vi "HMI Startup.vi"() -> ()   [LabVIEW 2019]
uses:
  <vilib>/Utility/sysdir.llb/System Directory Type.ctl
  <vilib>/NI/Current Value Table/Type Defs/Data Types.ctl
  <vilib>/NI/Current Value Table/Type Defs/Single Tag.ctl
  <vilib>/NI/STM/TCP/Read Meta Data (TCP Ref).vi
  <vilib>/NI/Current Value Table/DataTypes/Boolean_Write.vi
  <vilib>/NI/STM/TCP/Get Connection Reference (TCP).vi
  <vilib>/NI/Current Value Table/Type to Enum.vi
  <vilib>/NI/Current Value Table/DataTypes/Boolean_Type To Enum.vi
  <vilib>/NI/STM/TCP/Read Meta Data (TCP Clst).vi
  <vilib>/NI/STM/TCP/Write Message (TCP).vi
  <vilib>/NI/Current Value Table/FGVs/CVT Globals.vi
  <vilib>/NI/Current Value Table/FGVs/Tag Memory.vi
  <vilib>/NI/Current Value Table/Memory Block.vi
  <vilib>/NI/Current Value Table/DataTypes/Boolean_Memory Block.vi
  <vilib>/NI/Current Value Table/Current Value Table.lvlib
  <vilib>/NI/STM/NI STM.lvlib
panel:
  in  "Listbox":i32(listbox)=-1
  out "Sweep Time":dbl(graph)
  out "PLC Sweep Time":dbl
  out "Stop":bool
  out "PLC Firmware":string
  out "PLC Model":string
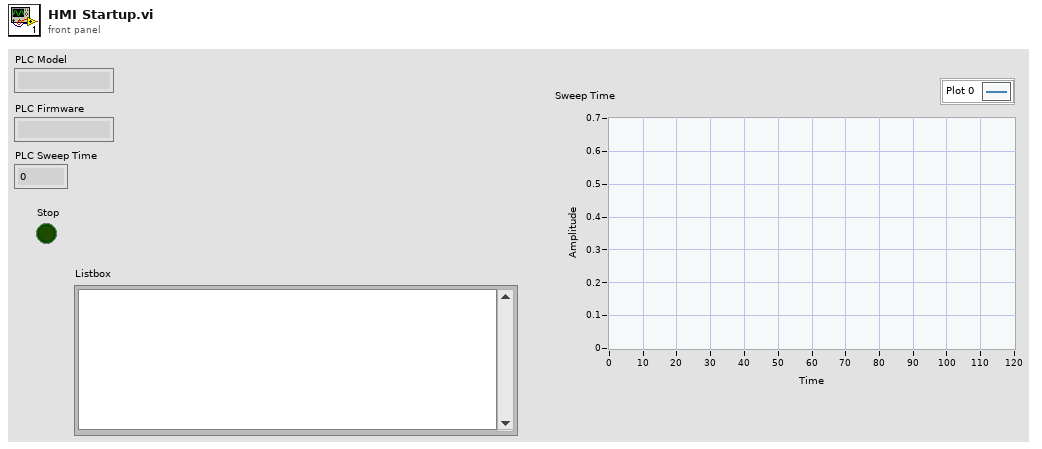
[diagram p1: front panel]
types:
  T1 = typedef "Current Value Table.lvlib/Single Tag.ctl" = cluster{"Data Type":T2, "Name":string, "Value":string, "Description":string}
  T2 = typedef "Current Value Table.lvlib/Data Types.ctl" = enum16{"Double", "Single", "I64", "I32", "I16", "I8", "U64", "U32", "U16", "U8", "String", "Boolean", "Array of U8", "Array of U16", "Array of U32", "Array of U64", "Array of I64", "Array of I32", "Array of I16", "Array of I8", "Array of Double", "Array of Single", "Array of Boolean", "Array of String"}
  T3 = typedef "System Directory Type.ctl" = i32
  T4 = typedef "tae_AlarmTagConfiguration.ctl" = cluster{"Name":string, "DataType":T5, "Alarm Configuration":T6}
  T5 = typedef "cvt_Data Types.ctl" = enum16{"Bool", "U8", "I32", "Double", "String", "Enum"}
  T6 = typedef "tae_AlarmConfiguration.ctl" = cluster{"Type":T7, "High Level":dbl, "Low Level":dbl, "Hysterisis":dbl, "Deadband":dbl}
  T7 = typedef "tae_AlarmType.ctl" = enum32{"Bool True", "Bool False", "Over Limit", "Under Limit", "Out-of-Range", "Enum Equal", "Enum Not Equal"}
  T8 = typedef "Current Value Table.lvlib/File Format.ctl" = cluster{"Tags":T1[], "Group Listings":T9[]}
  T9 = typedef "Current Value Table.lvlib/Tag Grouping set.ctl" = cluster{"Group":string, "Tag Names":string[]}
  T10 = typedef "NI STM.lvlib/TCP Connection Info.ctl" = cluster{"connection ID":refnum<k5>, "meta data":T11[]}
  T11 = typedef "NI STM.lvlib/MetaDataElement.ctl" = string
  T12 = typedef "tae_AlarmCommOut.ctl" = refnum<queue>
  T13 = typedef "tae_AlarmTagList.ctl" = T4[]
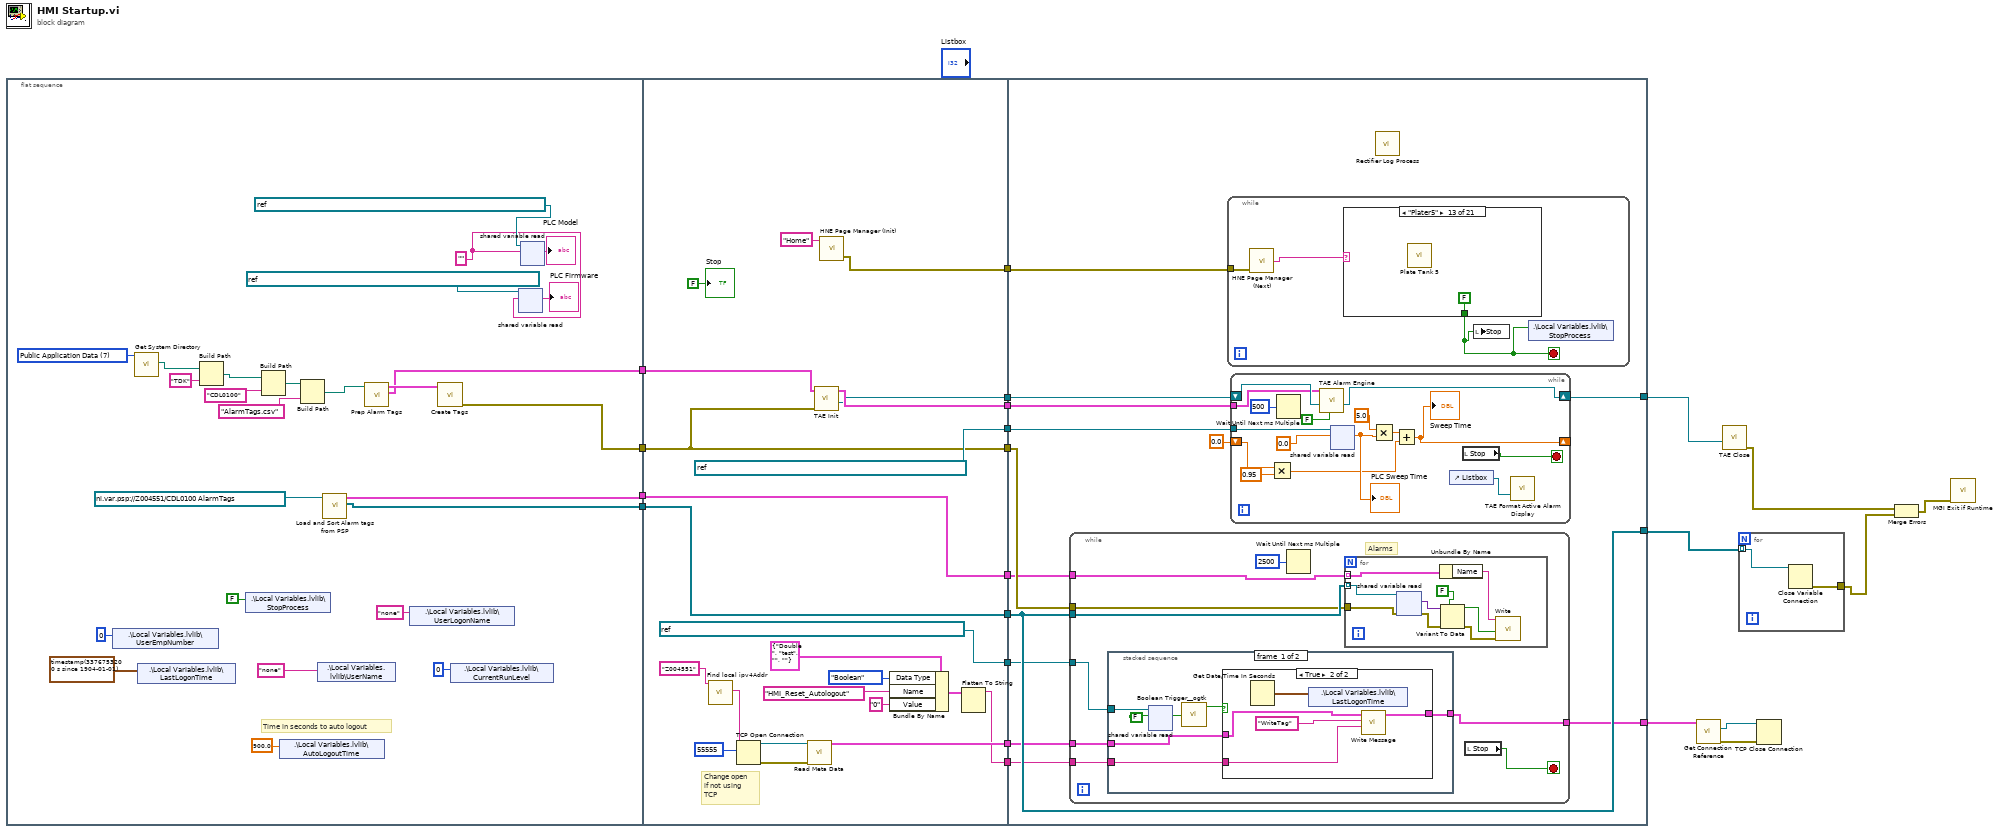
[diagram p0: block diagram]
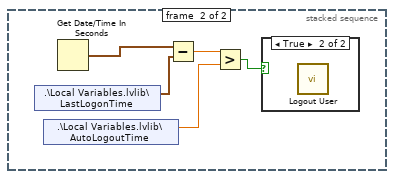
[diagram p3: hidden frame]
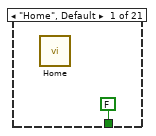
[diagram p5: hidden frame]
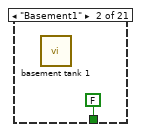
[diagram p6: hidden frame]
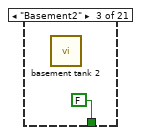
[diagram p7: hidden frame]
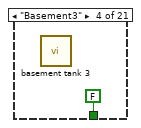
[diagram p8: hidden frame]
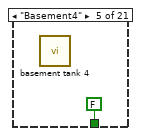
[diagram p9: hidden frame]
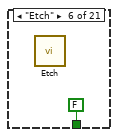
[diagram p10: hidden frame]
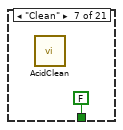
[diagram p11: hidden frame]
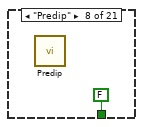
[diagram p12: hidden frame]
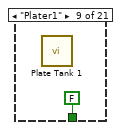
[diagram p13: hidden frame]
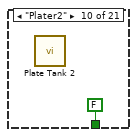
[diagram p14: hidden frame]
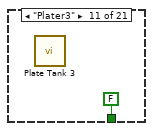
[diagram p15: hidden frame]
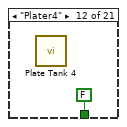
[diagram p16: hidden frame]
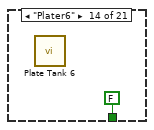
[diagram p17: hidden frame]
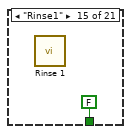
[diagram p18: hidden frame]
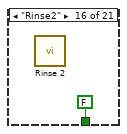
[diagram p19: hidden frame]
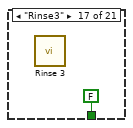
[diagram p20: hidden frame]
diagram:
  n1 = flat-sequence {
    tunnel: [w41] -> w19
    tunnel: [w39] -> w16
    tunnel: [w43] -> w14
    tunnel: [w42] -> w11
    tunnel: [w70] -> w22
    tunnel: [refnum<k21> "ni.var.psp://localhost/CDL0100 PLCSystem Tags/Sweep Time" ("shared variable refnum in")] -> w21
    tunnel: w19 -> [w68]
    tunnel: [w68] -> w18
    tunnel: w16 -> [w62]
    tunnel: [w67] -> w15
    tunnel: w14 -> [w67]
    tunnel: [w66] -> w13
    tunnel: [w65] -> w12
    tunnel: w11 -> [w63]
    tunnel: [w63] -> w10
    tunnel: [refnum<k21> "ni.var.psp://z004551/CDL0100 ReadWriteTags/HMI_Reset_Autologout" ("shared variable refnum in")] -> w6
    tunnel: [w55] -> w5
    tunnel: [w49] -> w4
    tunnel: w22 -> [w84]
    tunnel: w21 -> [w83]
    tunnel: [w82] -> w20
    tunnel: w18 -> [w81]
    tunnel: [w81] -> w17
    tunnel: w15 -> [w80]
    tunnel: w13 -> [w79]
    tunnel: w12 -> [w78]
    tunnel: w10 -> [w77]
    tunnel: w6 -> [w75]
    tunnel: w5 -> [w74]
    tunnel: w4 -> [w73]
    tunnel: [w72] -> w3
    frame #0 {
      w37 = T3 7 items=["User Home"=0, "User Desktop"=1, "User Documents"=2, "User Application Data"=3, "User Preferences"=4, "User Temporary"=5, "Public Documents"=6, "Public Application Data"=7, "Public Preferences"=8, "Public Cache"=13, "System Core Libraries"=9, "System Installed Libraries"=10, "Application Files"=11, "Boot Volume Root"=12] ("system directory type")
      w45 = ""
      # "Time in seconds to auto logout"
      n2 = shared-variable ".\\Local Variables.lvlib\\UserEmpNumber"(0 ("UserEmpNumber")) -> ()  [unwired: 1 in, 1 out]
      n3 = call <vilib>:"Get System Directory.vi"("system directory type"=w37) -> ("system directory"=w36:path)  [unwired: 10 in]
      n4 = shared-variable ".\\Local Variables.lvlib\\LastLogonTime"(timestamp(3376753200 s since 1904-01-01)) -> ()  [unwired: 1 in, 1 out]
      n5 = Build Path(base path=w36, name or relative path="TDK") -> (appended path=w34:path)
      n6 = shared-variable ".\\Local Variables.lvlib\\StopProcess"(FALSE ("StopProcess")) -> ()  [unwired: 1 in, 1 out]
      n7 = Build Path(base path=w34, name or relative path="CDL0100") -> (appended path=w32:path)
      n8 = shared-variable ".\\Local Variables.lvlib\\AutoLogoutTime"(900.0 ("AutoLogoutTime")) -> ()  [unwired: 1 in, 1 out]
      n9 = Build Path(base path=w32, name or relative path="AlarmTags.csv") -> (appended path=w30:path)
      n10 = shared-variable ".\\Local Variables.lvlib\\UserName"("none") -> ()  [unwired: 1 in, 1 out]
      n11 = call "Load and Sort Alarm tags from PSP.vi"("Refnum in"=refnum<k21> "ni.var.psp://Z004551/CDL0100 AlarmTags") -> ("Array 2"=w41:refnum<k21>[], "Array"=w42:T1[])  [unwired: 9 in]
      n12 = call "Prep Alarm Tags.vi"("Alarm Tag Description path"=w30) -> ("Alarm Array"=w39:T4[], "CVT Tags to Create"=w40:T8)  [unwired: 9 in]
      n13 = shared-variable ".\\Local Variables.lvlib\\UserLogonName"("none" ("UserLogonName")) -> ()  [unwired: 1 in, 1 out]
      n14 = call <vilib>:"Create Tags.vi"("CVT Tags to Create"=w40) -> ("error out"=w43:errorcluster)  [unwired: 10 in]
      n15 = shared-variable ".\\Local Variables.lvlib\\CurrentRunLevel"(0 ("CurrentRunLevel")) -> ()  [unwired: 1 in, 1 out]
      n16 = shared-variable-read(refnum<k21> "ni.var.psp://localhost/CDL0100 PLCSystem Tags/Firmware Version" ("shared variable refnum in"), w45) -> (→"PLC Firmware":string)  [unwired: 1 in, 3 out]
      n17 = shared-variable-read(refnum<k21> "ni.var.psp://localhost/CDL0100 PLCSystem Tags/Catalog Number" ("shared variable refnum in"), w45) -> (→"PLC Model":string)  [unwired: 1 in, 3 out]
    }
    frame #1 {
      # "Change open if not using TCP"
      n18 = call "Find local ipv4Addr.vi"("MachineToFind"="Z004551" ("Target IP Address")) -> ("name"=w56:string)  [unwired: 9 in, 1 out]
      n19 = TCP Open Connection(address=w56, remote port or service name=u16 55555 ("remote port")) -> (connection ID=w59:refnum<k5>, error out=w58:errorcluster)  [unwired: 1 in, 2 out]
      n20 = call-poly <vilib>:"Read Meta Data.vi"("error in"=w58, "connection ID"=w59) -> ("connection info out"=w55:T10)  [unwired: 7 in, 2 out]
      n21 = call <userlib>:"TAE Init.vi"("error in (no error)"=w67, "Alarm List"=w62) -> ("queue out"=w65:T12, "Alarm List"=w66:T13)  [unwired: 7 in, 1 out]
      n22 = call <userlib>:"HNE Page Manager (Init).vi"("Initial Page"="Home") -> ("error out"=w70:errorcluster)  [unwired: 4 in]
      n23 = Bundle By Name(cluster=T1 {"Data Type"=enum."Double", "Name"="test", "Value"="", "Description"=""} ("Tag"), "Data Type"=Data_Types."Boolean", "Name"="HMI_Reset_Autologout", "Value"="0") -> (w50:T1)
      n24 = Flatten To String(anything=w50) -> (data string=w49:string)  [unwired: 3 in, 2 out]
      "Stop" <- FALSE ("Stop")
    }
    frame #2 {
      n25 = while {
        tunnel: w81 -> [w91]
        tunnel: w80 -> [w90]
        tunnel: w77 -> [w89]
        tunnel: w75 -> [w88]
        tunnel: w74 -> [w87]
        tunnel: w73 -> [w86]
        tunnel: [w85] -> w72
        stop <- w93 stop-if-true
        # "Alarms"
        n26 = stacked-sequence {
          tunnel: w88 -> [w99 _]
          tunnel: w87 -> [w96 _]
          tunnel: w86 -> [w95 _]
          tunnel: [w94 _] -> w85
          frame #0 {
            n27 = shared-variable-read(w99, FALSE) -> (w98:bool)  [unwired: 1 in, 3 out]
            n28 = call <userlib>:"Boolean Trigger__ogtk.vi"("Boolean Input"=w98) -> ("Rising Edge"=w97:bool)  [unwired: 1 in, 1 out]
            n29 = case shown="True" w97 {
              tunnel: w96 -> [w101 w104]
              tunnel: w95 -> [_ w103]
              tunnel: [w101 w102] -> w94
              frame False {
              }
              frame True {
                n30 = Get Date/Time In Seconds() -> (seconds since 1Jan1904=w106:timestamp)
                n31 = shared-variable ".\\Local Variables.lvlib\\LastLogonTime"(w106) -> ()  [unwired: 1 in, 1 out]
                n32 = call-poly <vilib>:"Write Message.vi"("data"=w103, "name"="WriteTag", "connection info in"=w104) -> ("connection info out"=w102:T10)  [unwired: 7 in, 1 out]
              }
            }
          }
          frame #1 {
            n33 = shared-variable ".\\Local Variables.lvlib\\LastLogonTime"() -> (w109:timestamp)  [unwired: 1 in, 1 out]
            n34 = shared-variable ".\\Local Variables.lvlib\\AutoLogoutTime"() -> (w111:dbl)  [unwired: 1 in, 1 out]
            n35 = Get Date/Time In Seconds() -> (seconds since 1Jan1904=w108:timestamp)
            n36 = Subtract(x=w108, y=w109) -> (x-y=w110:dbl)
            n37 = Greater?(x=w110, y=w111) -> (0:w107:bool)
            n38 = case shown="True" w107 {
              frame False {
              }
              frame True {
                n39 = call "Logout User.vi"() -> ()  [unwired: 11 in, 1 out]
              }
            }
          }
        }
        n40 = Wait Until Next ms Multiple(millisecond multiple=u32 2500) -> ()  [unwired: 1 out]
        n41 = for {
          tunnel: w91 -> [w120] mode=indexing
          tunnel: w90 -> [w114]
          tunnel: w89 -> [w112] mode=indexing
          n42 = shared-variable-read(w120, w114) -> (w115:errorcluster, w119:variant)  [unwired: 2 out]
          n43 = Unbundle By Name(w112) -> ("Name"=w113:string)
          n44 = Variant To Data(error in=w115, type=FALSE, Variant=w119) -> (data=w117:bool, error out=w116:errorcluster)
          n45 = call-poly <vilib>:"Write.vi"("error in (no error)"=w116, "Value"=w117, "Tag Name"=w113) -> ()  [unwired: 8 in, 1 out]
        }
        n46 = local read "Stop"() -> (w93:bool)
      }
      n47 = while {
        tunnel: w84 -> [w139]
        stop <- w137 stop-if-true
        n48 = call <userlib>:"HNE Page Manager (Next).vi"("error in (no error)"=w139) -> ("Next Page"=w138:string)  [unwired: 3 in, 1 out]
        n49 = case shown="\"Plater5\"" w138 {
          tunnel: [FALSE FALSE FALSE FALSE FALSE FALSE FALSE FALSE FALSE FALSE FALSE FALSE FALSE FALSE FALSE FALSE FALSE FALSE FALSE FALSE TRUE] -> w137
          frame "Home", Default {
            n50 = call "Home.vi"() -> ()  [unwired: 12 in]
          }
          frame "Basement1" {
            n51 = call "basement tank 1.vi"() -> ()  [unwired: 12 in]
          }
          frame "Basement2" {
            n52 = call "basement tank 2.vi"() -> ()  [unwired: 12 in]
          }
          frame "Basement3" {
            n53 = call "basement tank 3.vi"() -> ()  [unwired: 12 in]
          }
          frame "Basement4" {
            n54 = call "basement tank 4.vi"() -> ()  [unwired: 12 in]
          }
          frame "Etch" {
            n55 = call "Etch.vi"() -> ()  [unwired: 12 in]
          }
          frame "Clean" {
            n56 = call "AcidClean.vi"() -> ()  [unwired: 12 in]
          }
          frame "Predip" {
            n57 = call "Predip.vi"() -> ()  [unwired: 12 in]
          }
          frame "Plater1" {
            n58 = call "Plate Tank 1.vi"() -> ()  [unwired: 12 in]
          }
          frame "Plater2" {
            n59 = call "Plate Tank 2.vi"() -> ()  [unwired: 12 in]
          }
          frame "Plater3" {
            n60 = call "Plate Tank 3.vi"() -> ()  [unwired: 12 in]
          }
          frame "Plater4" {
            n61 = call "Plate Tank 4.vi"() -> ()  [unwired: 12 in]
          }
          frame "Plater5" {
            n62 = call "Plate Tank 5.vi"() -> ()  [unwired: 12 in]
          }
          frame "Plater6" {
            n63 = call "Plate Tank 6.vi"() -> ()  [unwired: 12 in]
          }
          frame "Rinse1" {
            n64 = call "Rinse 1.vi"() -> ()  [unwired: 12 in]
          }
          frame "Rinse2" {
            n65 = call "Rinse 2.vi"() -> ()  [unwired: 12 in]
          }
          frame "Rinse3" {
            n66 = call "Rinse 3.vi"() -> ()  [unwired: 12 in]
          }
          frame "Rinse4" {
            n67 = call "Rinse 4.vi"() -> ()  [unwired: 12 in]
          }
          frame "Dryer" {
            n68 = call "Dryer.vi"() -> ()  [unwired: 12 in]
          }
          frame "LockOut" {
            n69 = call "LockOut.vi"() -> ()  [unwired: 12 in]
          }
          frame "Exit" {
          }
        }
        n70 = local write "Stop"(w137) -> ()
        n71 = shared-variable ".\\Local Variables.lvlib\\StopProcess"(w137) -> ()  [unwired: 1 in, 1 out]
      }
      n72 = while {
        tunnel: w83 -> [w134]
        shift-right: [w130] -> w82
        shift-left: w78 -> [w131]
        tunnel: w79 -> [w129]
        shift-right: [w121] -> _
        shift-left: 0.0 -> [w127]
        stop <- w136 stop-if-true
        n73 = Multiply(x=w127, y=0.95) -> (x*y=w122:dbl)
        n74 = Wait Until Next ms Multiple(millisecond multiple=u32 500) -> ()  [unwired: 1 out]
        n75 = call <userlib>:"TAE Alarm Engine.vi"("Alarm Logging?"=FALSE, "AE_CommIn"=w131, "Alarm List"=w129) -> ("Alarm queue out"=w130:T12)  [unwired: 6 in, 2 out]
        n76 = shared-variable-read(w134, 0.0) -> (w125:dbl)  [unwired: 1 in, 3 out]
        "PLC Sweep Time" <- w125
        n77 = Multiply(x=5.0, y=w125) -> (x*y=w123:dbl)
        n78 = Add(x=w123, y=w122) -> (x+y=w121:dbl)
        "Sweep Time" <- w121
        n79 = control-ref of="Listbox"() -> (w128:refnum<vi>)
        n80 = local read "Stop"() -> (w136:bool)
        n81 = call <userlib>:"TAE Format Active Alarm Display.vi"("List Box Ref"=w128) -> ()  [unwired: 14 in, 1 out]
      }
      n82 = call "Rectifier Log Process.vi"() -> ()  [unwired: 12 in]
    }
  }
  n83 = call-poly <vilib>:"Get Connection Reference.vi"("connection info in"=w3) -> ("error out"=w1:errorcluster, "connection ID out"=w2:refnum<k5>)  [unwired: 1 in, 8 out]
  n84 = call <userlib>:"TAE Close.vi"("Alarm queue out"=w20) -> ("error out"=w9:errorcluster)  [unwired: 10 in]
  n85 = for {
    tunnel: w17 -> [w162] mode=indexing
    tunnel: [w161] -> w8
    n86 = Close Variable Connection(11:w162) -> (0:w161:errorcluster)  [unwired: 1 in]
  }
  n87 = TCP Close Connection(connection ID=w2, error in (no error)=w1) -> ()  [unwired: 3 out]
  n88 = Merge Errors(w9, w8) -> (w7:errorcluster)
  n89 = call <userlib>:"MGI Exit if Runtime.vi"("Error In (Dependency Only)"=w7) -> ()  [unwired: 11 in]
